vi "MTM2_putSample_axialActuatorPositionAbsoluteEncoderPositionMeasured.vi"(8 "error in (no error)":errorcluster, 11 "axialActuatorPositionAbsoluteEncoderPositionMeasured_Ctl":T1={"axialEncoderPositionMeasured[72]"=[0.0, 0.0, 0.0, 0.0, 0.0, 0.0, 0.0, 0.0, 0.0, 0.0, 0.0, 0.0, 0.0, 0.0, 0.0, 0.0, 0.0, 0.0, 0.0, 0.0, 0.0, 0.0, 0.0, 0.0, 0.0, 0.0, 0.0, 0.0, 0.0, 0.0, 0.0, 0.0, 0.0, 0.0, 0.0, 0.0, 0.0, 0.0, 0.0, 0.0, 0.0, 0.0, 0.0, 0.0, 0.0, 0.0, 0.0, 0.0, 0.0, 0.0, 0.0, 0.0, 0.0, 0.0, 0.0, 0.0, 0.0, 0.0, 0.0, 0.0, 0.0, 0.0, 0.0, 0.0, 0.0, 0.0, 0.0, 0.0, 0.0, 0.0, 0.0, 0.0]}) -> (0 "error out":errorcluster, 2 "function return":i32, 3 "axialActuatorPositionAbsoluteEncoderPositionMeasured_Ctl out":T1)   [LabVIEW 2018, in "SALLV_MTM2.lvlib"]
doc: "int MTM2_shm_putSample_axialActuatorPositionAbsoluteEncoderPositionMeasuredLV(MTM2_axialActuatorPositionAbsoluteEncoderPositionMeasuredLV *axialActuatorPositionAbsoluteEncoderPositionMeasured_Ctl );"
uses:
  SALLV_MTM2.lvlib
  DataTypes/axialActuatorPositionAbsoluteEncoderPositionMeasured.ctl
  SALLV_MTM2.so
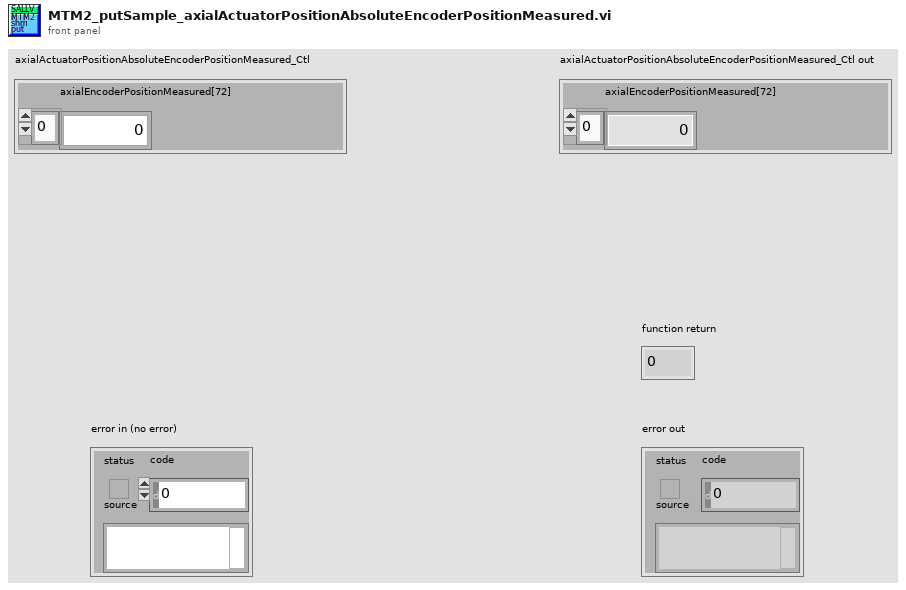
[diagram p1: front panel]
types:
  T1 = typedef "SALLV_MTM2.lvlib/axialActuatorPositionAbsoluteEncoderPositionMeasured.ctl" = cluster{"axialEncoderPositionMeasured[72]":dbl[]}
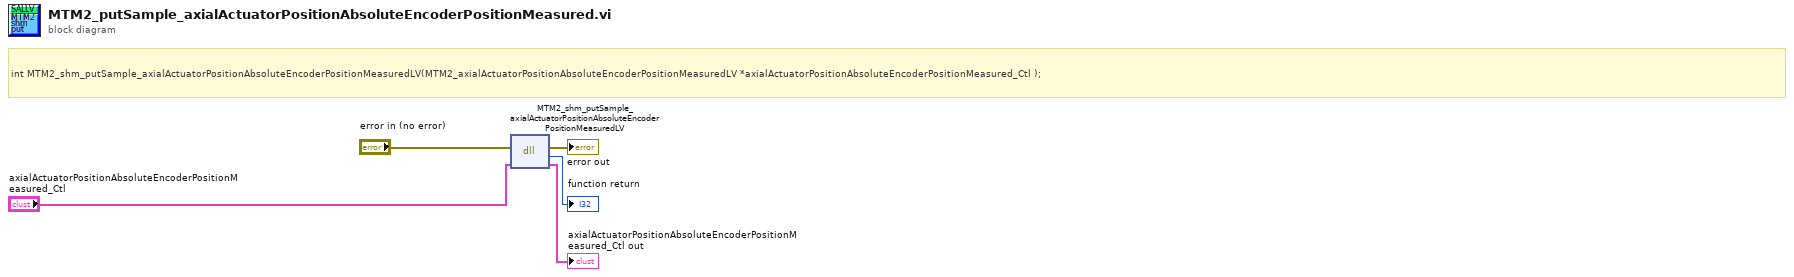
[diagram p0: block diagram]
diagram:
  # "int MTM2_shm_putSample_axialActuatorPositionAbsoluteEncoderPositionMeasuredLV(MTM2_axialActuatorPositionAbsoluteEncoderPositionMeasuredLV *axialActuatorPositionAbsoluteEncoderPositionMeasured_Ctl );"
  n1 = dll-call lib="home/ttsai/Document/salApiMTM2/SALLV_MTM2/SALLV_MTM2.*" fn="MTM2_shm_putSample_axialActuatorPositionAbsoluteEncoderPositionMeasuredLV"(error in="error in (no error)", "axialActuatorPositionAbsoluteEncoderPositionMeasured_Ctl"="axialActuatorPositionAbsoluteEncoderPositionMeasured_Ctl") -> (error out=→"error out":errorcluster, →"function return":i32, "axialActuatorPositionAbsoluteEncoderPositionMeasured_Ctl"=→"axialActuatorPositionAbsoluteEncoderPositionMeasured_Ctl out":T1)  [unwired: 2 in, 1 out]
